vi "Initialize.vi"(8 "error in":errorcluster, 9 "Number of Channels":u32=1, 10 "Plugin Name":string, 11 "Control Mode in":refnum<class "Control Mode.lvclass">) -> (0 "error out":errorcluster, 3 "Control Mode out":refnum<class "Control Mode.lvclass">)   [LabVIEW 2023, in "Control Mode.lvclass"]
uses:
  Control Mode.lvclass
  Mode.ctl
  Control Mode.lvclass/Control Mode.ctl
  <vilib>/ADAS Replay HIL/Channels/Tag Wrapper/Polymorphic/Open Consumer Tag (U32).vi
  <vilib>/ADAS Replay HIL/Channels/Tag Wrapper/Polymorphic/Set Default Value (U32).vi
  <vilib>/ADAS Replay HIL/Channels/Tag Wrapper/Polymorphic/Open Consumer Tag (U32).vi/bacb721e-673a-491a-accd-959f2e1f334e.vi
  <vilib>/ADAS Replay HIL/Channels/Tag Wrapper/Polymorphic/Set Default Value (U32).vi/228e99de-6fcf-414d-86fc-dc277c7b351f.vi
  <vilib>/ADAS Replay HIL/Channels/Tag Wrapper/Polymorphic/Open Consumer Tag (U32).vi/bacb721e-673a-491a-accd-959f2e1f334e.vi/c28b0ead-42ad-4072-80a2-aca7f2bd7ce3.vi
  <vilib>/ADAS Replay HIL/Channels/Tag Wrapper/Polymorphic/Set Default Value (U32).vi/228e99de-6fcf-414d-86fc-dc277c7b351f.vi/4bc1c15b-36ab-481f-b8dd-c64075ce723a.vi
  <vilib>/ADAS Replay HIL/AdasHilServices/AdasHilServices Fill In Error Info Ex.vi
  <vilib>/ADAS Replay HIL/Channels/Tag Wrapper/Tag Wrapper.lvlib
  Utilities/Utilities.lvlib
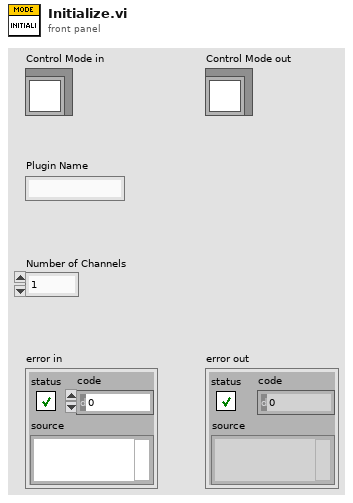
[diagram p1: front panel]
types:
  T1 = typedef "Control Mode.lvclass/Mode.ctl" = u32
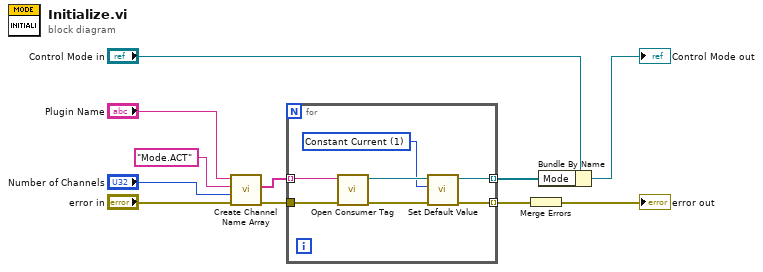
[diagram p0: block diagram]
diagram:
  n1 = call "Create Channel Name Array.vi"("error in"="error in", "Number of Channels"="Number of Channels", "Channel Format String"="Mode.ACT" ("Channel Name"), "Plugin Name"="Plugin Name") -> ("error out"=w10:errorcluster, "Channel Names"=w11:string[])  [unwired: 6 in]
  n2 = for {
    tunnel: w11 -> [w18] mode=indexing
    tunnel: [w13] -> w4 mode=indexing
    tunnel: w10 -> [w17]
    tunnel: [w14] -> w8 mode=indexing
    w12 = T1 1 items=["Constant Current"=1, "Constant Voltage"=2, "Battery Emulator"=100, "Fuel Cell Emulator"=101] ("Ring")
    n3 = call-poly <vilib>:"Open Consumer Tag.vi"("error in"=w17, "Channel Name"=w18) -> ("error out"=w15:errorcluster, "ADAS HIL Channel"=w16:refnum<k21>)  [unwired: 8 in]
    n4 = call-poly <vilib>:"Set Default Value.vi"("error in"=w15, "Default Value"=w12, "ADAS HIL Channel in"=w16) -> ("error out"=w14:errorcluster, "ADAS HIL Channel out"=w13:refnum<k21>)  [unwired: 7 in]
  }
  n5 = Merge Errors(w8) -> (→"error out":errorcluster)
  n6 = Bundle By Name(cluster="Control Mode in", "Mode"=w4) -> (→"Control Mode out":refnum<class "Control Mode.lvclass">)
